vi "AssignSignals.vi"(8 "Error in":errorcluster, 11 "DevicesAndSignals":T1) -> (0 "Error out":errorcluster, 3 "DevicesAndSignals":T1)   [LabVIEW 2016]
doc: "Assigns the settings of the given signals to the physical signal of the according device."
uses:
  C:/Users/CL/Desktop/ZcDAQprj0811/ZcDAQprj/Modules/DAQ-Device/Hardware Drivers/QX/HBM LabVIEW Driver/DLLs/Hbm.Api.Common.dll
  DLLs/Hbm.Api.Common.dll
  C:/Users/CL/Desktop/ZcDAQprj0811/ZcDAQprj/Modules/DAQ-Device/Hardware Drivers/QX/HBM LabVIEW Driver/DLLs/Hbm.Api.LabVIEW.dll
  DLLs/Hbm.Api.LabVIEW.dll
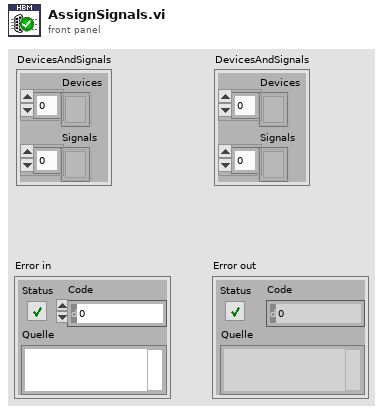
[diagram p1: front panel]
types:
  T1 = cluster{"Devices":refnum<k24>[], "Signals":refnum<k24>[]}
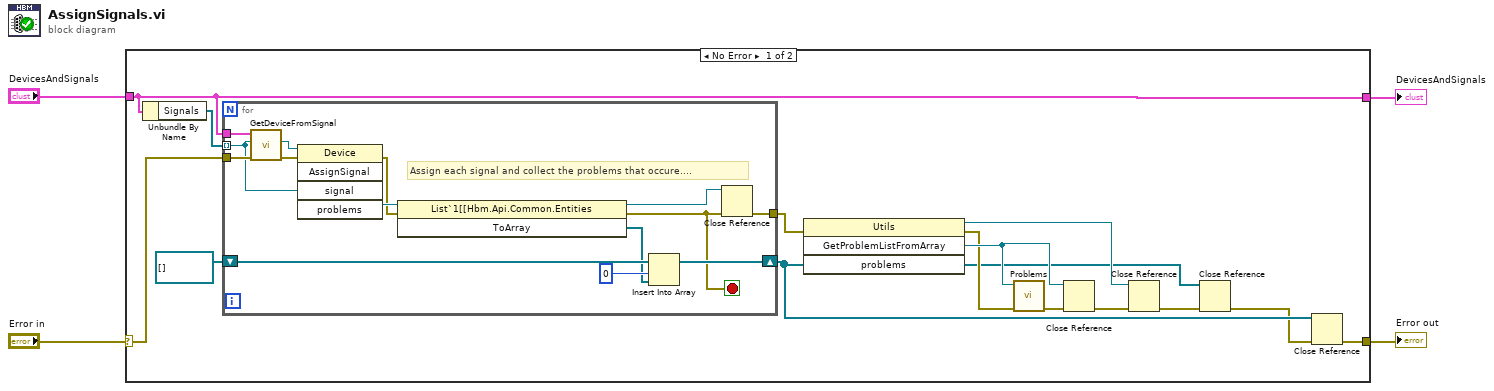
[diagram p0: block diagram]
diagram:
  n1 = case shown="No Error" "Error in" {
    selector: "Error in" -> [w16 w35]
    tunnel: "DevicesAndSignals" -> [w11 w34]
    tunnel: [w5 w35] -> w3
    tunnel: [w11 w34] -> w1
    frame No Error {
      n2 = Unbundle By Name(w11) -> ("Signals"=w19:refnum<k24>[])
      n3 = for {
        tunnel: w19 -> [w22] mode=indexing
        tunnel: w11 -> [w33]
        tunnel: w16 -> [w32]
        shift-right: [w29] -> w9
        shift-left: refnum<k24>[] [] -> [w28]
        tunnel: [w21] -> w17
        stop <- w24 stop-if-true
        # "Assign each signal and collect the problems that occure...."
        n4 = call "GetDeviceFromSignal.vi"("Error in"=w32, "Signal"=w22, "DevicesAndSignals"=w33) -> ("Error out"=w30:errorcluster, "Device"=w31:refnum<k24>)  [unwired: 6 in, 1 out]
        n5 = invoke on="Methodenknoten" class="Device" method="AssignSignal"(reference=w31, error in=w30, "signal"=w22) -> (error out=w25:errorcluster, "problems"=w26:refnum<k24>)  [unwired: 2 in, 3 out]
        n6 = invoke on="Methodenknoten" class="List`1[[Hbm.Api.Common.Entities" method="ToArray"(reference=w26, error in=w25) -> (reference out=w23:refnum<k24>, error out=w24:errorcluster, "ToArray"=w20:refnum<k24>[])  [unwired: 1 in]
        n7 = Insert Into Array(array=w28, index=0 ("Index"), new element=w20) -> (w29:refnum<k24>[])
        n8 = Close Reference(reference=w23, error in (no error)=w24) -> (error out=w21:errorcluster)
      }
      n9 = invoke on="Methodenknoten" class="Utils" method="GetProblemListFromArray"(error in=w17, "problems"=w9) -> (reference out=w12:refnum<k24>, error out=w10:errorcluster, "GetProblemListFromArray"=w14:refnum<k24>, "problems"=w6:refnum<k24>[])  [unwired: 2 in]
      n10 = call "Problems.vi"("Error in"=w10, "Problems"=w14) -> ("Error out"=w15:errorcluster)  [unwired: 9 in]
      n11 = Close Reference(reference=w14, error in (no error)=w15) -> (error out=w13:errorcluster)
      n12 = Close Reference(reference=w12, error in (no error)=w13) -> (error out=w7:errorcluster)
      n13 = Close Reference(reference=w6, error in (no error)=w7) -> (error out=w8:errorcluster)
      n14 = Close Reference(reference=w9, error in (no error)=w8) -> (error out=w5:errorcluster)
    }
    frame Error {
    }
  }
  "DevicesAndSignals" <- w1
  "Error out" <- w3
